vi "产生一个周期性随机噪声信号.vi"() -> ()   [LabVIEW 2018]
uses:
  <vilib>/measure/NI_MABase.lvlib
panel:
  in  "reset signal":bool caption="重置信号"
  in  "sampling info":cluster{"Fs":dbl, "#s":dbl}={"Fs"=1000.0, "#s"=1000.0} caption="采样信息" {"Fs" format="%.2p"}
  in  "停止":bool
  out "波形图":waveform(dbl)(graph)
  in  "seed":i32=-1 caption="种子"
  in  "spectral amplitude":dbl=1.0 caption="频谱幅值" format="%.2p"
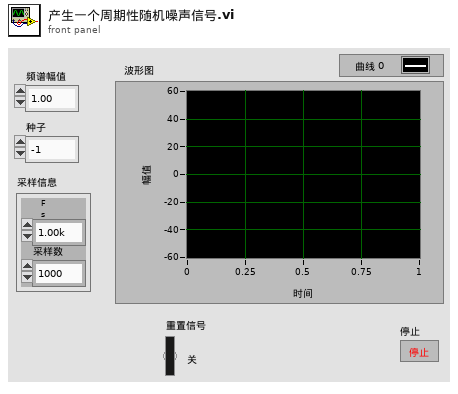
[diagram p1: front panel]
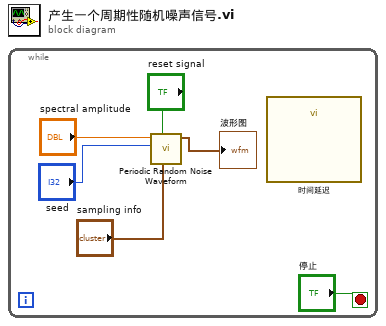
[diagram p0: block diagram]
diagram:
  n1 = while {
    stop <- "停止" stop-if-true
    n2 = call <vilib>:"Periodic Random Noise Waveform.vi"("sampling info"="sampling info", "reset signal"="reset signal", "seed"="seed", "spectral amplitude"="spectral amplitude") -> ("signal out"=→"波形图":waveform(dbl))  [unwired: 6 in, 1 out]
    n3 = call "时间延迟"() -> ()  [unwired: 11 in, 1 out]
  }
